vi "Refresh Rooms Status.vi"(0 "Hotel Management Tool Model in":refnum<class "Hotel Management Tool Model.lvclass">, 5 "Rooms List":T2[](array[typedef]), 7 "Room Size Details":T1[](array[typedef]), 11 "error in (no error)":errorcluster) -> (4 "Hotel Management Tool Model out":refnum<class "Hotel Management Tool Model.lvclass">, 15 "error out":errorcluster)   [LabVIEW 2023, in "Hotel Management Tool Model.lvlib" / "Hotel Management Tool Model.lvclass"]
uses:
  Hotel Management Tool Model.lvclass
  Central Data Manager/Central Data Manager/Room Details.ctl
  Central Data Manager/Central Data Manager/Room Occupancy Status.ctl
  Central Data Manager/Central Data Manager/Guest Details.ctl
  Central Data Manager/Central Data Manager/Room Size Details.ctl
  Hotel Management Tool Model.lvclass/Hotel Management Tool Model.ctl
  Rooms Manager Model/Rooms Manager Model Messages/Refresh Rooms Status Msg/Refresh Rooms Status Msg.lvclass/Refresh Rooms Status Msg.ctl
  <vilib>/ActorFramework/Message Enqueuer/Message Enqueuer.lvclass/Message Enqueuer.ctl
  <vilib>/ActorFramework/Message Enqueuer/Enqueue.vi
  Rooms Manager Model/Rooms Manager Model Messages/Refresh Rooms Status Msg/Refresh Rooms Status Msg.lvclass
  C:/Program Files/National Instruments/LabVIEW 2023/vi.lib/ActorFramework/Message/Message.lvclass
  <vilib>/ActorFramework/Message Priority Queue/Priority Enqueue.vi
  Central Data Manager/Central Data Manager/Central Data Manager.lvclass
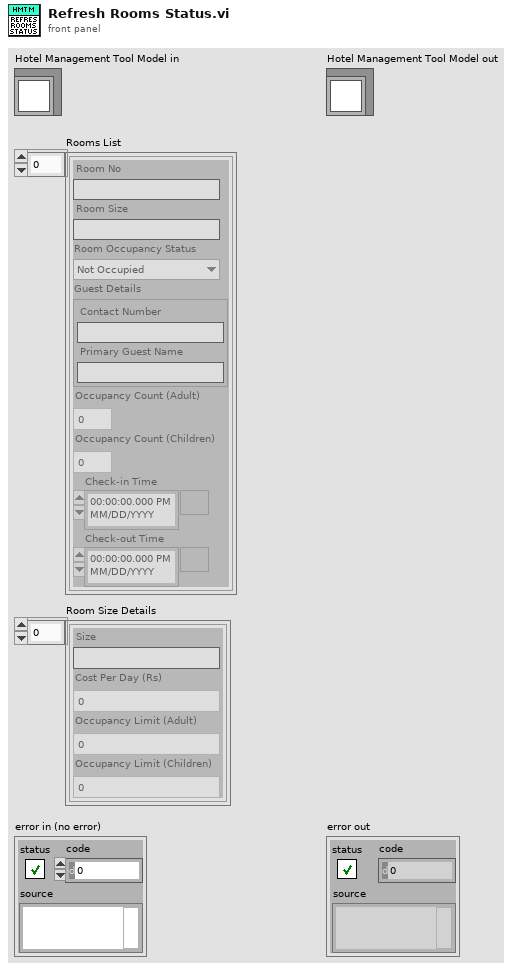
[diagram p1: front panel]
types:
  T1 = typedef "Central Data Manager.lvlib/Central Data Manager.lvclass/Room Size Details.ctl" = cluster{"Size":string, "Cost Per Day (Rs)":u32, "Occupancy Limit (Adult)":u32, "Occupancy Limit (Children)":u32}
  T2 = typedef "Central Data Manager.lvlib/Central Data Manager.lvclass/Room Details.ctl" = cluster{"Room No":string, "Room Size":string, "Room Occupancy Status":T3, "Guest Details":T4, "Occupancy Count (Adult)":u32, "Occupancy Count (Children)":u32, "Check-in Time":timestamp, "Check-out Time":timestamp}
  T3 = typedef "Central Data Manager.lvlib/Central Data Manager.lvclass/Room Occupancy Status.ctl" = enum16{"Not Occupied", "Occupied", "Under Maintainance", "Not Servicable"}
  T4 = typedef "Central Data Manager.lvlib/Central Data Manager.lvclass/Guest Details.ctl" = cluster{"Contact Number":string, "Primary Guest Name":string}
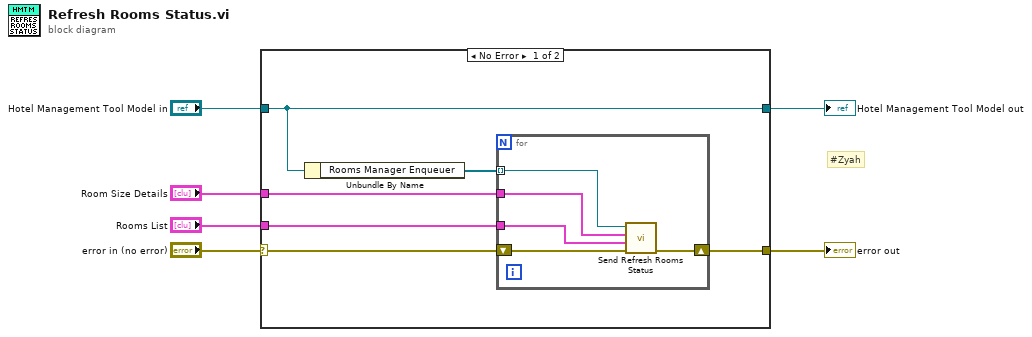
[diagram p0: block diagram]
diagram:
  # "#Zyah"
  n1 = case shown="No Error" "error in (no error)" {
    selector: "error in (no error)" -> [w12 w19]
    tunnel: [w11 w19] -> w5
    tunnel: [w8 w18] -> w3
    tunnel: "Hotel Management Tool Model in" -> [w8 w18]
    tunnel: "Room Size Details" -> [w10 _]
    tunnel: "Rooms List" -> [w9 _]
    frame No Error {
      n2 = Unbundle By Name(w8) -> ("Rooms Manager Enqueuer"=w7:refnum<class "Message Enqueuer.lvclass">[])
      n3 = for {
        tunnel: w10 -> [w15]
        tunnel: w9 -> [w14]
        shift-right: [w16] -> w11
        shift-left: w12 -> [w17]
        tunnel: w7 -> [w13] mode=indexing
        n4 = call "Send Refresh Rooms Status.vi"("error in (no error)"=w17, "Rooms List"=w14, "Room Size Details"=w15, "Message Enqueuer"=w13) -> ("error out"=w16:errorcluster)  [unwired: 6 in, 1 out]
      }
    }
    frame Error {
    }
  }
  "error out" <- w5
  "Hotel Management Tool Model out" <- w3
